vi "FloodFill.vi"() -> ()   [LabVIEW 2023, in "2021_12.lvclass"]
uses:
  2021_12.lvclass
  <userlib>/_OpenG.lib/string/string.llb/openg_string.lvlib
panel:
  out "product":i32
  out "Array":i32[](array[numeric])
  out "x >= y?":bool[][](array[boolean])
  out "PixelsFound":cluster{"x":i32, "y":i32}[](array[cluster])
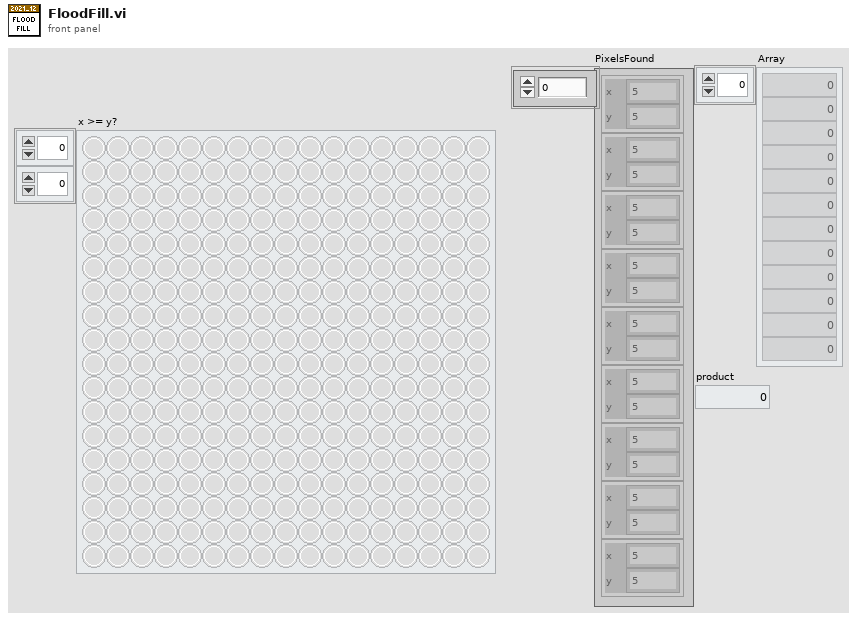
[diagram p1: front panel]
types:
  T1 = cluster{"PixelsFound":cluster{"x":i32, "y":i32}[]}[]
  T2 = cluster{"PixelsFound":cluster{"x":i32, "y":i32}[]}
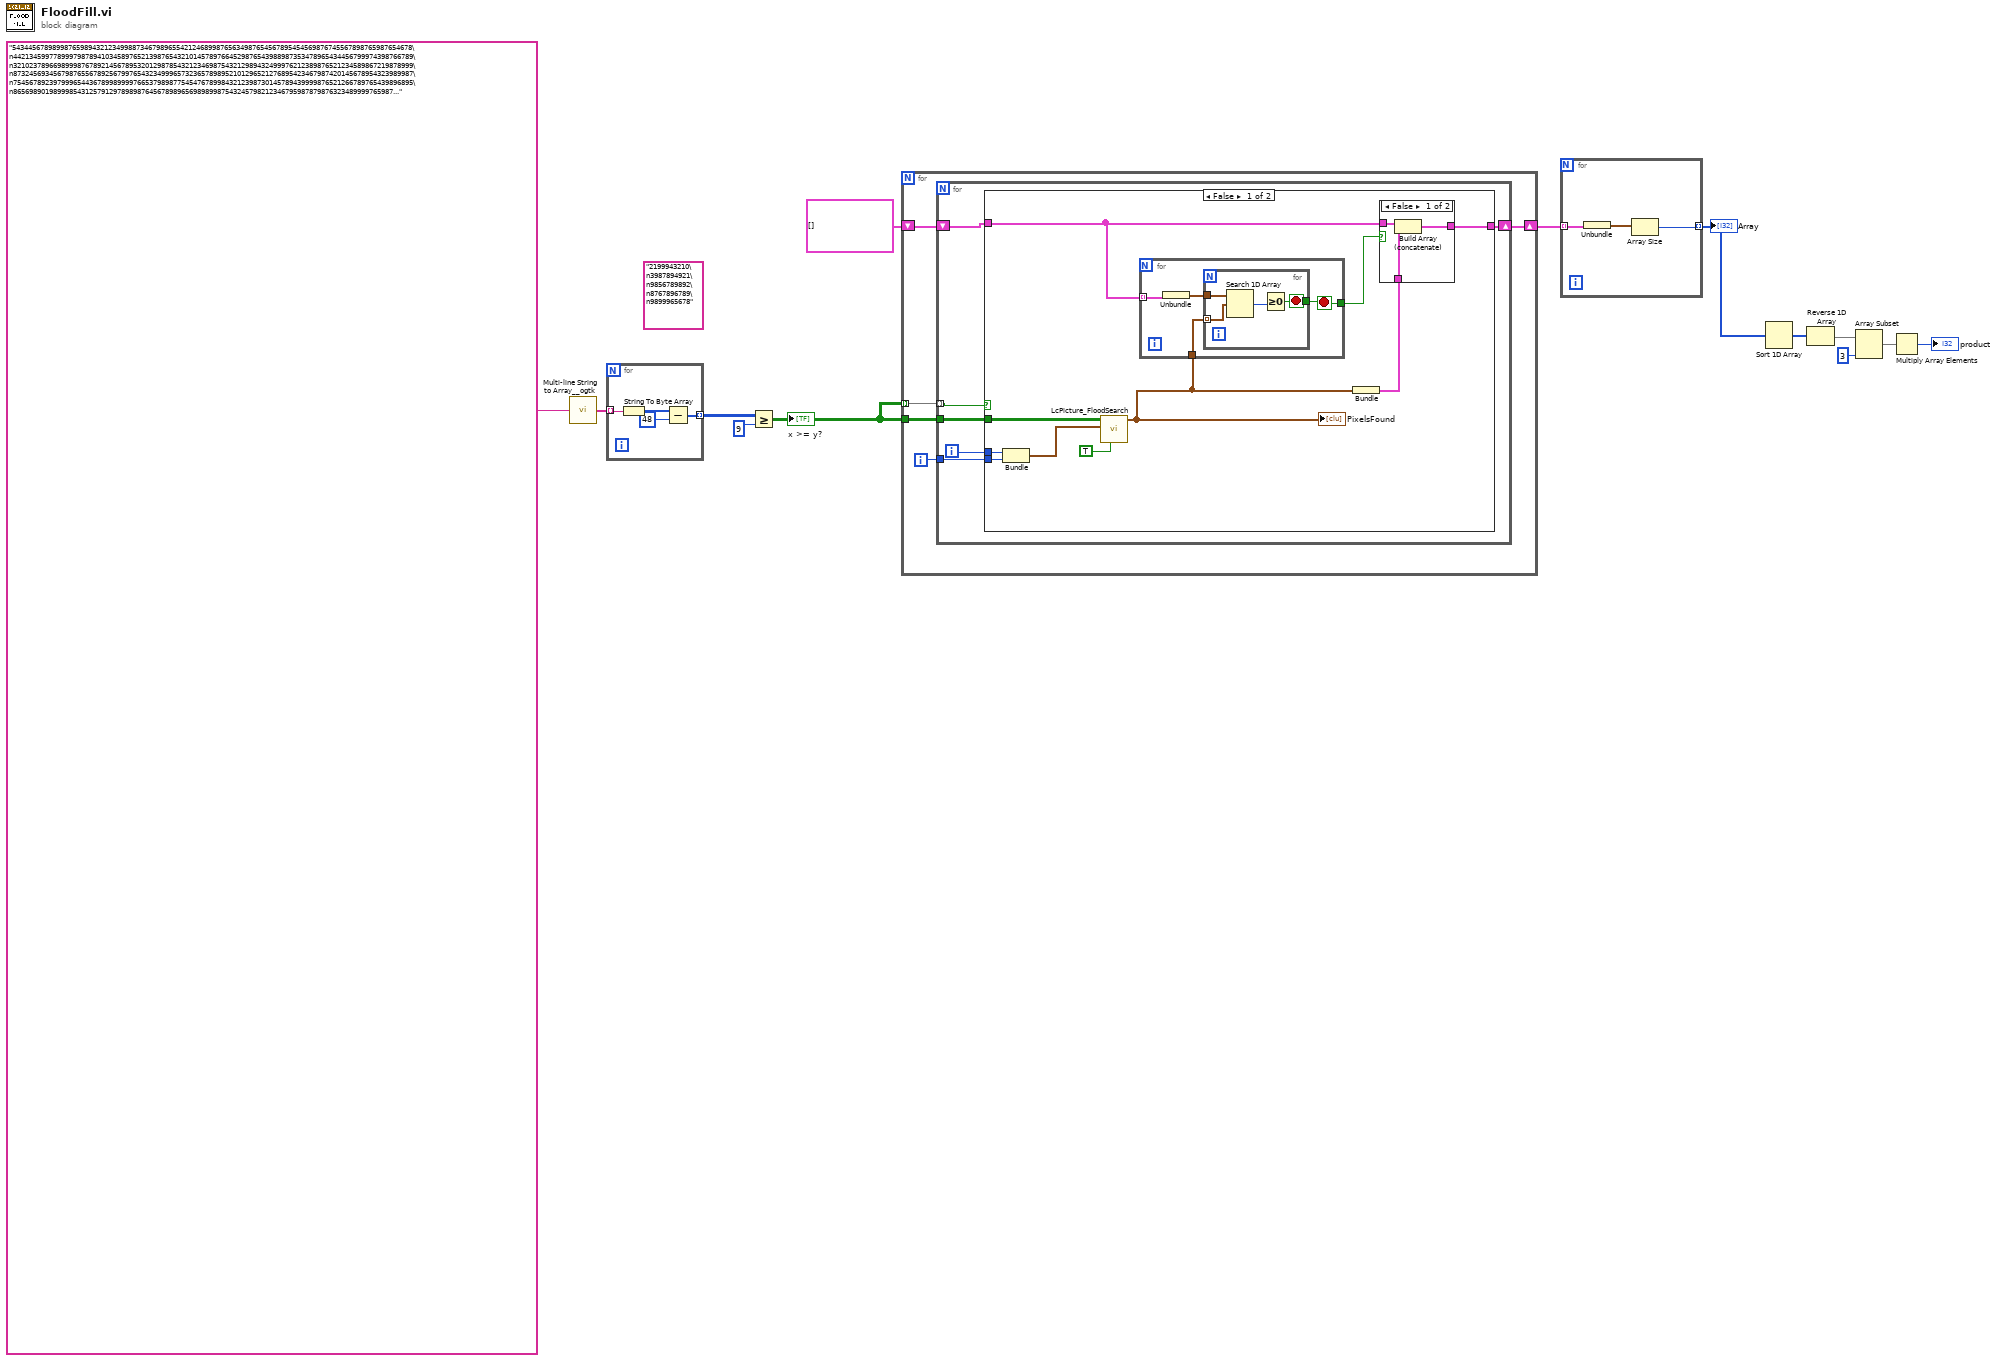
[diagram p0: block diagram]
diagram:
  (unwired) "2199943210\n3987894921\n9856789892\n8767896789\n9899965678"
  n1 = call <userlib>:"Multi-line String to Array__ogtk.vi"("string"="5434456789899876598943212349988734679896554212468998765634987654567895454569876745567898765987654678\n4421345997789997987894103458976521398765432101457897664529876543988987353478965434456799974398766789\n3210237896698999876789214567895320129878543212346987543212989432499976212389876521234589867219878999\n8732456934567987655678925679976543234999657323657898952101296521276895423467987420145678954323989987\n7545678923979996544367899899997665379898775454767899843212398730145789439999876521266789765439896895\n86569890198999854312579129789898764567898965698989987543245798212346795987879876323489999765987...") -> ("lines"=w12:string[])
  n2 = for {
    tunnel: w12 -> [w17] mode=indexing
    tunnel: [w14] -> w11 mode=indexing
    n3 = String To Byte Array(string=w17) -> (unsigned byte array=w15:u8[])
    n4 = Subtract(x=w15, y=u8 48) -> (x-y=w14:u8[])
  }
  n5 = Greater Or Equal?(x=w11, y=u8 9) -> (x >= y?=w9:bool[][])
  "x >= y?" <- w9
  n6 = for {
    tunnel: w9 -> [w22]
    tunnel: w9 -> [w21] mode=indexing
    shift-right: [w18] -> w7
    shift-left: T1 [] -> [w19]
    i -> [w20]
    n7 = for {
      tunnel: w22 -> [w28]
      tunnel: w21 -> [w27] mode=indexing
      tunnel: w20 -> [w25]
      shift-right: [w23] -> w18
      shift-left: w19 -> [w24]
      i -> [w26]
      n8 = case shown="False" w27 {
        tunnel: w28 -> [w37 _]
        tunnel: w26 -> [w36 _]
        tunnel: w25 -> [w35 _]
        tunnel: w24 -> [w31 w51]
        tunnel: [w33 w51] -> w23
        frame False {
          n9 = Bundle(w36, w35) -> (w34:cluster{i32, i32})  [unwired: 1 in]
          n10 = call <userlib>:"LcPicture_FloodSearch.vi"("4 (T) or 8 (F)"=TRUE, "Start Position"=w34, "DataIn"=w37) -> ("PixelsFound"=w30:cluster{"x":i32, "y":i32}[])  [unwired: 5 in, 3 out]
          "PixelsFound" <- w30
          n11 = for {
            tunnel: w31 -> [w46] mode=indexing
            tunnel: w30 -> [w45]
            tunnel: [w43] -> w29
            stop <- w43 stop-if-true
            n12 = Unbundle(w46) -> ("PixelsFound"=w44:cluster{"x":i32, "y":i32}[])
            n13 = for {
              tunnel: w45 -> [w49] mode=indexing
              tunnel: w44 -> [w50]
              tunnel: [w47] -> w43
              stop <- w47 stop-if-true
              n14 = Search 1D Array(1D array=w50, element=w49) -> (index of element=w48:i32)  [unwired: 1 in]
              n15 = Greater Or Equal To 0?(x=w48) -> (x >= 0?=w47:bool)
            }
          }
          n16 = Bundle("PixelsFound"=w30) -> (w32:T2)  [unwired: 1 in]
          n17 = case shown="False" w29 {
            tunnel: [w41 w42] -> w33
            tunnel: w32 -> [w40 _]
            tunnel: w31 -> [w39 w42]
            frame False {
              n18 = Build Array (concatenate)(w39, w40) -> (w41:T1)
            }
            frame True {
            }
          }
        }
        frame True {
        }
      }
    }
  }
  n19 = for {
    tunnel: w7 -> [w54] mode=indexing
    tunnel: [w52] -> w6 mode=indexing
    n20 = Unbundle(w54) -> ("PixelsFound"=w53:cluster{"x":i32, "y":i32}[])
    n21 = Array Size(array=w53) -> (size(s)=w52:i32)
  }
  "Array" <- w6
  n22 = Sort 1D Array(array=w6) -> (sorted array=w5:i32[])
  n23 = Reverse 1D Array(array=w5) -> (reversed array=w4:i32[])
  n24 = Array Subset(array=w4, length=3) -> (w2:i32[])  [unwired: 1 in]
  n25 = Multiply Array Elements(1:w2) -> (0:→"product":i32)
